vi "normalizeRobotAngle.vi"(8 "error in (no error)":errorcluster, 10 "signal":dbl, 11 "Utilities in":refnum<class "Utilities.lvclass">) -> (0 "error out":errorcluster, 2 "signal 2":dbl, 3 "Utilities out":refnum<class "Utilities.lvclass">)   [LabVIEW 2020, in "Utilities.lvclass"]
uses:
  Utilities.lvclass
  <vilib>/ptbypt/NI_PtbyPt.lvlib
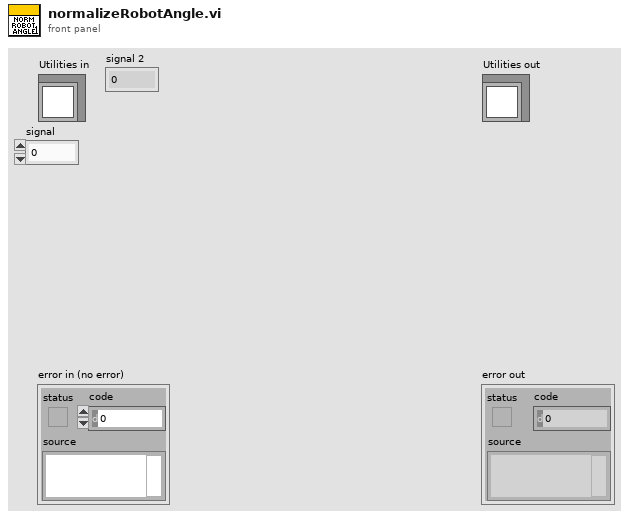
[diagram p1: front panel]
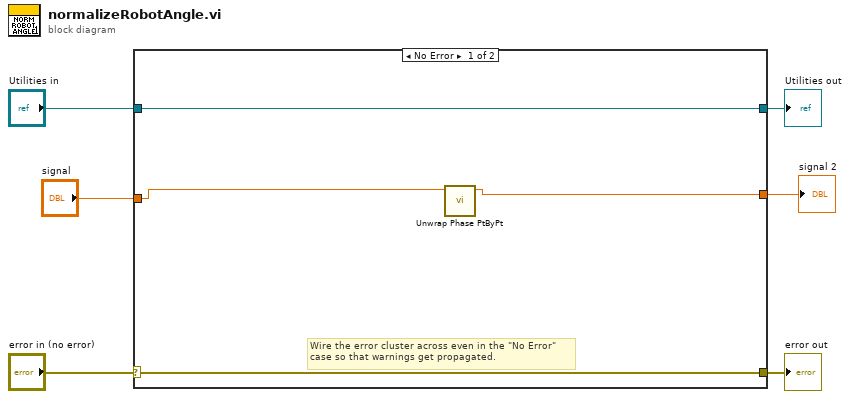
[diagram p0: block diagram]
diagram:
  n1 = case shown="No Error" "error in (no error)" {
    selector: "error in (no error)" -> [w9 w12]
    tunnel: [w9 w12] -> w5
    tunnel: [w10 w11] -> w3
    tunnel: "Utilities in" -> [w10 w11]
    tunnel: "signal" -> [w8 _]
    tunnel: [w7 _] -> w1
    frame No Error {
      # "Wire the error cluster across even in the \"No Error\"\ncase so that warnings get propagated."
      n2 = call <vilib>:"Unwrap Phase PtByPt.vi"("phase"=w8) -> ("unwrapped phase"=w7:dbl)  [unwired: 10 in]
    }
    frame Error {
    }
  }
  "error out" <- w5
  "Utilities out" <- w3
  "signal 2" <- w1
